vi "Update Obj Position.vi"(8 "error in (no error)":errorcluster, 11 "Boolean Object Position in":refnum<class "Boolean Object Position.lvclass">) -> (0 "error out":errorcluster, 3 "Boolean Object Position out":refnum<class "Boolean Object Position.lvclass">)   [LabVIEW 2018, in "Boolean Object Position.lvclass"]
uses:
  Boolean Object Position.lvclass
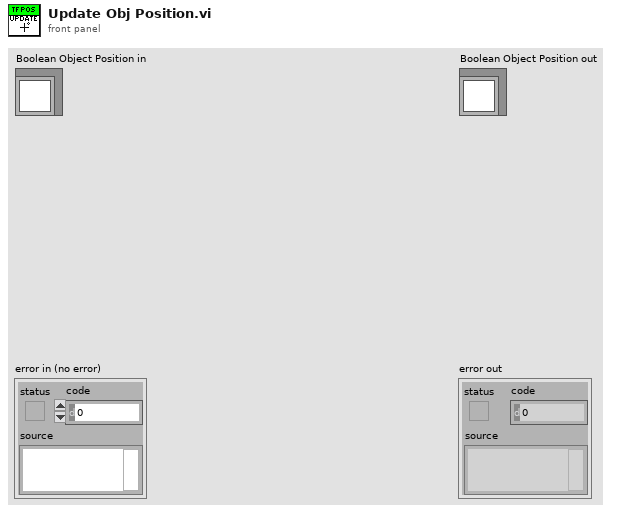
[diagram p1: front panel]
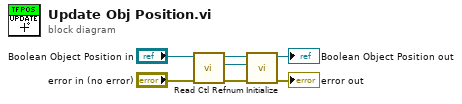
[diagram p0: block diagram]
diagram:
  n1 = call-dynamic "Read Ctl Refnum.vi"("error in (no error)"="error in (no error)", "Pane Object Position in"="Boolean Object Position in") -> ("error out"=w4:errorcluster, "Ctl Refnum"=w1:refnum<vi>, "Pane Object Position out"=w2:refnum<class "Boolean Object Position.lvclass">)  [unwired: 7 in]
  n2 = call-dynamic "Initialize.vi"("error in (no error)"=w4, "Ctl Refnum"=w1, "Boolean Object Position in"=w2) -> ("error out"=→"error out":errorcluster, "Boolean Object Position out"=→"Boolean Object Position out":refnum<class "Boolean Object Position.lvclass">)  [unwired: 7 in]
